vi "Read Refine.vi"(8 "error in (no error)":errorcluster, 11 "Point Correspondence Params in":refnum<class "Point Correspondence Params.lvclass">) -> (0 "error out":errorcluster, 2 "Refine":bool=TRUE, 3 "Point Correspondence Params out":refnum<class "Point Correspondence Params.lvclass">)   [LabVIEW 2020, in "toolkit.lvlib" / "Point Correspondence Params.lvclass"]
doc: "Read Refine.\n\nSee https://pointclouds.org/documentation/classpcl_1_1registration_1_1_correspondence_rejector_sample_consensus.html for more information."
uses:
  Point Correspondence Params.lvclass
  Point Correspondence Params.lvclass/Point Correspondence Params.ctl
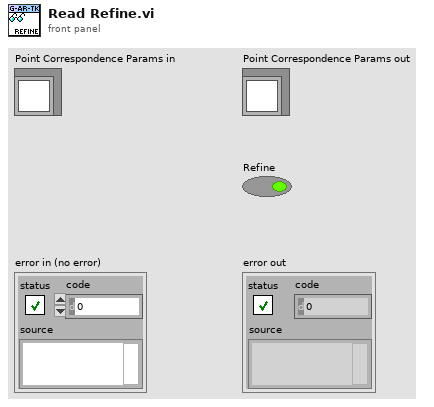
[diagram p1: front panel]
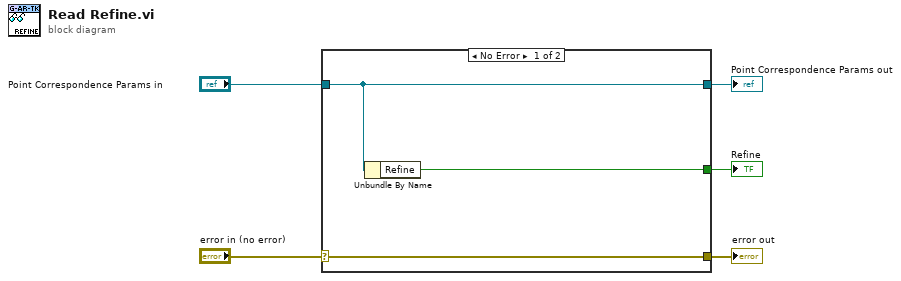
[diagram p0: block diagram]
diagram:
  n1 = case shown="No Error" "error in (no error)" {
    selector: "error in (no error)" -> [w8 w9]
    tunnel: [w8 w9] -> w4
    tunnel: [w7 w10] -> w2
    tunnel: "Point Correspondence Params in" -> [w7 w10]
    tunnel: [w6 _] -> w1
    frame No Error {
      n2 = Unbundle By Name(w7) -> ("Refine"=w6:bool)
    }
    frame Error {
    }
  }
  "error out" <- w4
  "Point Correspondence Params out" <- w2
  "Refine" <- w1
